vi "PAQ_BIN_IndexRangeCheck.vi"(8 "error in (no error)":errorcluster, 9 "Stop":timestamp, 10 "Start":timestamp, 11 "TimeStamps":T1(array[cluster])) -> (0 "error out":errorcluster, 1 "Tables":string[](array[string]), 3 "Sequences":i32[](array[numeric]))   [LabVIEW 2020, in "Sgraph_lib_V1.lvlib" / "DBAL-BIN.lvclass"]
doc: "Check if the IDX index content fall within the range of the Start and Stop time"
uses:
  DBAL-BIN.lvclass
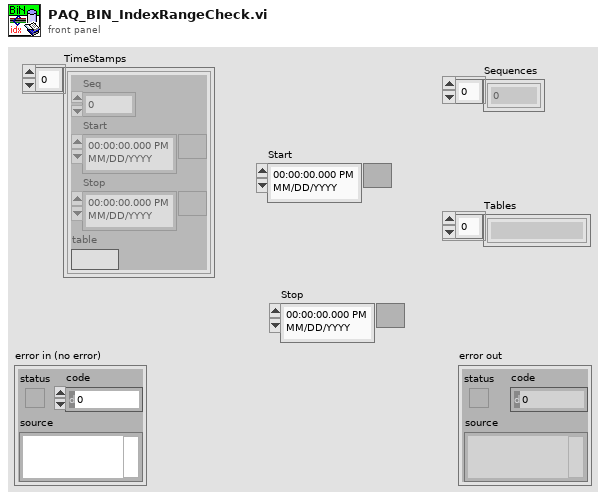
[diagram p1: front panel]
types:
  T1 = cluster{"Seq":i32, "Start":timestamp, "Stop":timestamp, "table":string}[]
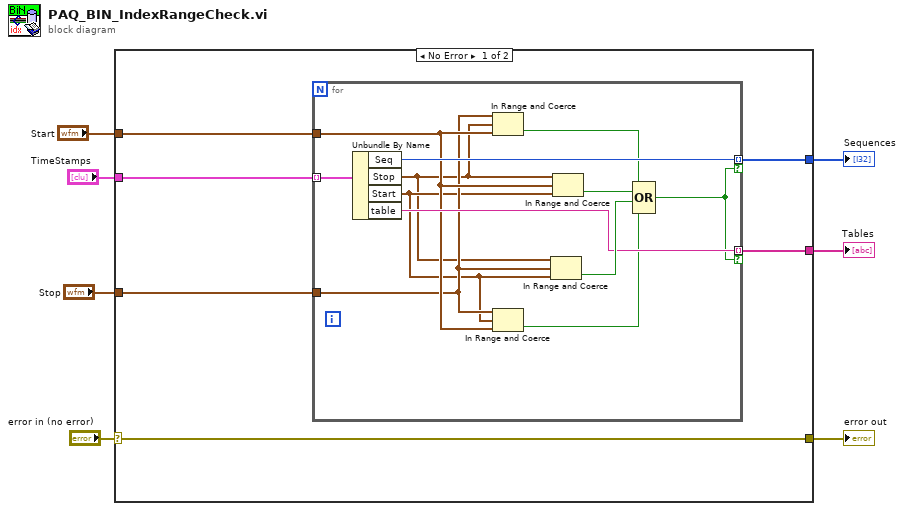
[diagram p0: block diagram]
diagram:
  n1 = case shown="No Error" "error in (no error)" {
    selector: "error in (no error)" -> [w8 w26]
    tunnel: "TimeStamps" -> [w13 _]
    tunnel: "Start" -> [w12 _]
    tunnel: "Stop" -> [w11 _]
    tunnel: [w10 _] -> w3
    tunnel: [w9 _] -> w2
    tunnel: [w8 w26] -> w1
    frame No Error {
      n2 = for {
        tunnel: w13 -> [w25] mode=indexing
        tunnel: w12 -> [w20]
        tunnel: [w24] -> w10 mode=indexing if=w14
        tunnel: w11 -> [w19]
        tunnel: [w21] -> w9 mode=indexing if=w14
        n3 = Unbundle By Name(w25) -> ("Seq"=w24:i32, "Stop"=w15:timestamp, "Start"=w16:timestamp, "table"=w21:string)
        n4 = In Range and Coerce(upper limit=w19, x=w15, lower limit=w20) -> (In Range?=w18:bool)  [unwired: 1 out]
        n5 = In Range and Coerce(upper limit=w19, x=w16, lower limit=w20) -> (In Range?=w17:bool)  [unwired: 1 out]
        n6 = In Range and Coerce(upper limit=w15, x=w19, lower limit=w16) -> (In Range?=w23:bool)  [unwired: 1 out]
        n7 = In Range and Coerce(upper limit=w15, x=w20, lower limit=w16) -> (In Range?=w22:bool)  [unwired: 1 out]
        n8 = Compound Arithmetic op=OR(w18, w22, w23, w17) -> (w14:bool)
      }
    }
    frame Error {
    }
  }
  "error out" <- w1
  "Sequences" <- w3
  "Tables" <- w2
